vi "main_v1.vi"() -> ()   [LabVIEW 2020]
uses:
  <vilib>/Analysis/Matrix/Datatypes/RealMatrix.ctl
  C:/Program Files (x86)/National Instruments/LabVIEW 2020/examples/Instrument IO/Serial/support/Serial - Settings.ctl
  C:/Program Files (x86)/National Instruments/LabVIEW 2020/examples/Instrument IO/Serial/support/Serial - XON-XOFF Characters.ctl
  C:/Program Files (x86)/National Instruments/LabVIEW 2020/examples/Instrument IO/Serial/support/Serial - ASCII Characters.ctl
  <vilib>/Platform/TimedLoop/XDataNode/timing_clust.ctl
  <vilib>/Platform/TimedLoop/XDataNode/nitl_modes.ctl
  <vilib>/Platform/TimedLoop/XDataNode/wakeup.ctl
  <vilib>/Instr/_visa.llb/VISA Configure Serial Port (Instr).vi
  <vilib>/platform/TimedLoop/XDataNode/XDataNode.xnode
  <vilib>/Platform/TimedLoop/XDataNode/XDNodeRunTimeDep.lvlib
  <vilib>/Analysis/Matrix/NI_Matrix.lvlib
panel:
  out "Angle Plot":cluster{"Y":dbl[], "Y":dbl[]}[](graph)
  out "Z_GYRO":dbl(graph)
  out "Y_GYRO":dbl(graph)
  out "X_GYRO":dbl(graph)
  out "Z_ACC":dbl(graph)
  out "X_ACC":dbl(graph)
  out "Y_ACC":dbl(graph)
  out "Angular velocity after filtering":dbl
  out "pitch after filtering in degrees":dbl
  in  "Stop":bool
  in  "Read Count":u32=1000
  in  "?":bool
  in  "Termination Character":u8=10 format="%.0x"
  in  "End Write on Termination Character?":bool=TRUE
  in  "VISA resource name":refnum<visa-resource-name>="COM1"
  in  "XON/XOFF Characters":T1={"XON"=enum."DC1", "XOFF"=enum."DC3"}
  in  "Serial Settings":T3={"baud rate"=9600, "data bits"=8, "parity"=enum."None", "stop bits"=10, "flow control"=0} {"flow control" items=["None"=0, "XON/XOFF"=1, "RTS/CTS"=2, "DTR/DSR"=4]; "stop bits" items=["1.0"=10, "1.5"=15, "2.0"=20]; "data bits" min=5 max=8 step=1; "baud rate" items=["75"=75, "110"=110, "134"=134, "150"=150, "300"=300, "600"=600, "1200"=1200, "1800"=1800, "2400"=2400, "4800"=4800, "7200"=7200, "9600"=9600, "14400"=14400, "19200"=19200, "28800"=28800, "38400"=38400, "56000"=56000, "57600"=57600, "115200"=115200, "128000"=128000, "230400"=230400]}
  in  "End Read on Termination Character?":bool=TRUE
  out "Steady State Kalman Predictor Gain matrix":T4=[[-7.62521027355318e-05, 0.01032332398776421], [0.031126923690244213, -7.313941036650737e-06]]
  out "H Matrix":T4=[[0.0, 1.0], [1.0, 0.0]]
  out "G Matrix":T4=[[0.0001, -5e-09], [0.0, 0.0001]]
  out "F  Matrix":T4=[[1.0, -0.0001], [0.0, 1.0]]
  out "Q'=GQG' (Q scalar =1)":T4=[[1.0000000025e-08, -5e-13], [-5e-13, 1e-08]]
  out "State Predicted Estimate X^(k+1/k)":dbl[](array[numeric])=[-1.7557452195435928, 0.08364774980311916]
  out "Angular Velocity for Pitch":dbl(graph)
  out "Pitch Angle in degrees":dbl(graph)
  in  "Kalman Filter -> SWITCH OFF":bool=TRUE
  out "Raw X Gyro Velocity":dbl=-1.8293611669128778
  out "Raw accelerometer angle in degrees":dbl=-1.8293611669128778
  in  "X degrees  offset trim angle":dbl=-2.4999999999999982 min=-20.0 max=20.0 step=0.1
  in  "X offset trim gyro velocity":i16=60
  in  "Y offset trim gyro velocity":i16=-244
  out "Z_Acc":dbl=22.0 format="%.2f"
  out "Y_Acc":dbl=22.0 format="%.2f"
  out "X_Acc":dbl=22.0 format="%.2f"
  out "Z_Gyro_Rate":dbl=22.0 format="%.2f"
  out "X_Gyro_rate":dbl=22.0 format="%.2f"
  out "Y_Gyro_Rate":dbl=22.0 format="%.2f"
  # "Steady State Kalman Filter"
  # "-Prakhar Goel"
  # "Kalman Matrices"
  # "Serial Settings"
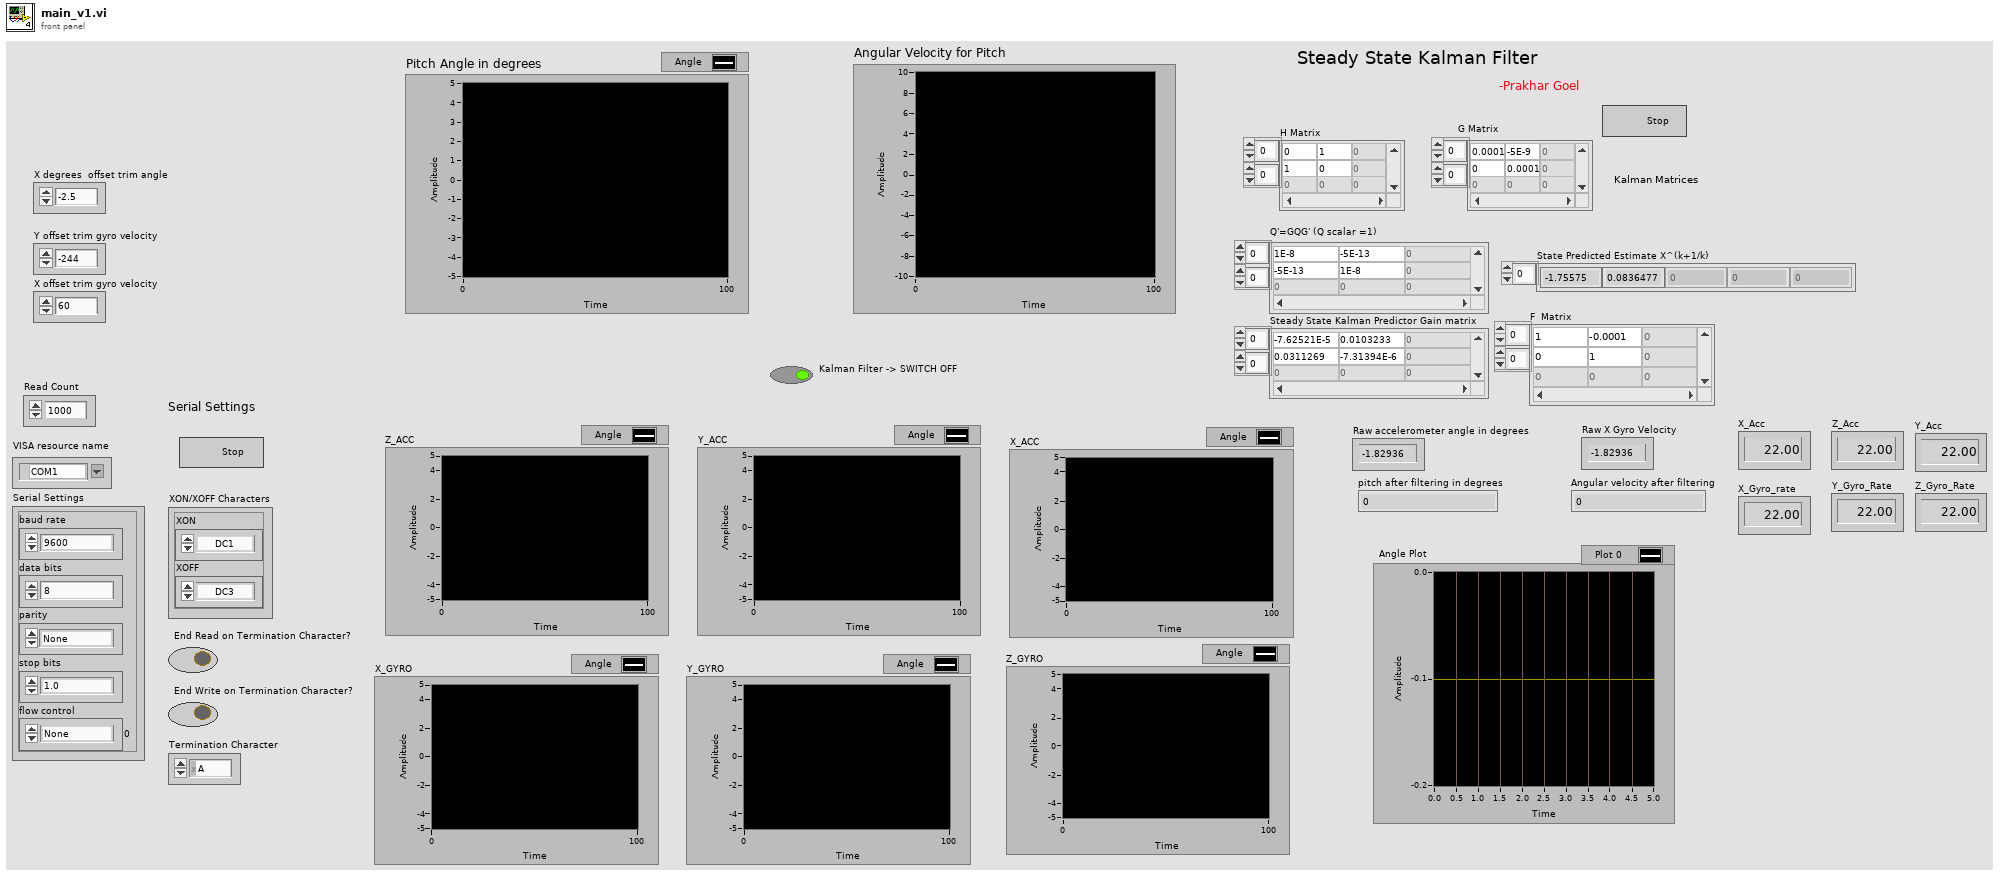
[diagram p1: front panel]
types:
  T1 = typedef "Serial - XON-XOFF Characters.ctl" = cluster{"XON":T2, "XOFF":T2}
  T2 = typedef "Serial - ASCII Characters.ctl" = enum16{"NUL", "SOH", "STX", "ETX", "EOT", "ENQ", "ACK", "BEL", "BS", "HT", "LF", "VT", "FF", "CR", "SO", "SI", "DLE", "DC1", "DC2", "DC3", "DC4", "NAK", "SYN", "ETB", "CAN", "EM", "SUB", "ESC", "FS", "GS", "RS", "US", "SP", "!", "\"", "#", "$", "%", "&", "'", "(", ")", "*", "+", ",", "- (-)", ".", "/", "0", "1", "2", "3", "4", "5", "6", "7", "8", "9", ":", ";", "<", "=", ">", "?", "@", "A", "B", "C", "D", "E", "F", "G", "H", "I", "J", "K", "L", "M", "N", "O", "P", "Q", "R", "S", "T", "U", "V", "W", "X", "Y", "Z", "[", "\\", "]", "^", "_", "`", "a", "b", "c", "d", "e", "f", "g", "h", "i", "j", "k", "l", "m", "n", "o", "p", "q", "r", "s", "t", "u", "v", "w", "x", "y", "z", "{", "|", "}", "~"}
  T3 = typedef "Serial - Settings.ctl" = cluster{"baud rate":u32, "data bits":u16, "parity":enum16{"None", "Odd", "Even", "Mark", "Space"}, "stop bits":u16, "flow control":u16}
  T4 = typedef "NI_Matrix.lvlib/RealMatrix.ctl" = dbl[][]
  T5 = typedef "XDNodeRunTimeDep.lvlib/timing_clust.ctl" = cluster{"Expected End [f-1]":u64, "Actual End [f-1]":u64, "Finished Late? [f-1]":bool, "Expected End [i-1]":u64, "Actual End [i-1]":u64, "Finished Late? [i-1]":bool, "Expected Start [i]":u64, "Actual Start [i]":u64, "Expected Start [f]":u64, "Actual Start [f]":u64, "Source Name":string, "Structure Name":string, "Period":i64, "Deadline":i64, "Offset":i64, "Start":i64, "Priority":i32, "Timeout":i32, "Mode":T6, "Wakeup Reason":T7, "Error":errorcluster, "Source Type":string, "Secondary Source Type":string, "Global End Time":u64, "Global Start Time":u64, "Frame Duration":u64, "Iteration Duration":u64, "Assigned CPU":i32, "I/O Scan Engine Mode":u32}
  T6 = typedef "XDNodeRunTimeDep.lvlib/nitl_modes.ctl" = enum32{"No Change", "Process missed periods, maintain original phase", "Discard missed periods, maintain original phase", "Process missed periods, ignore original phase", "Discard missed periods, ignore original phase"}
  T7 = typedef "XDNodeRunTimeDep.lvlib/wakeup.ctl" = enum32{"Normal", "Aborted", "Asynchronous wakeup", "Timing source error", "Timed loop error", "Timeout"}
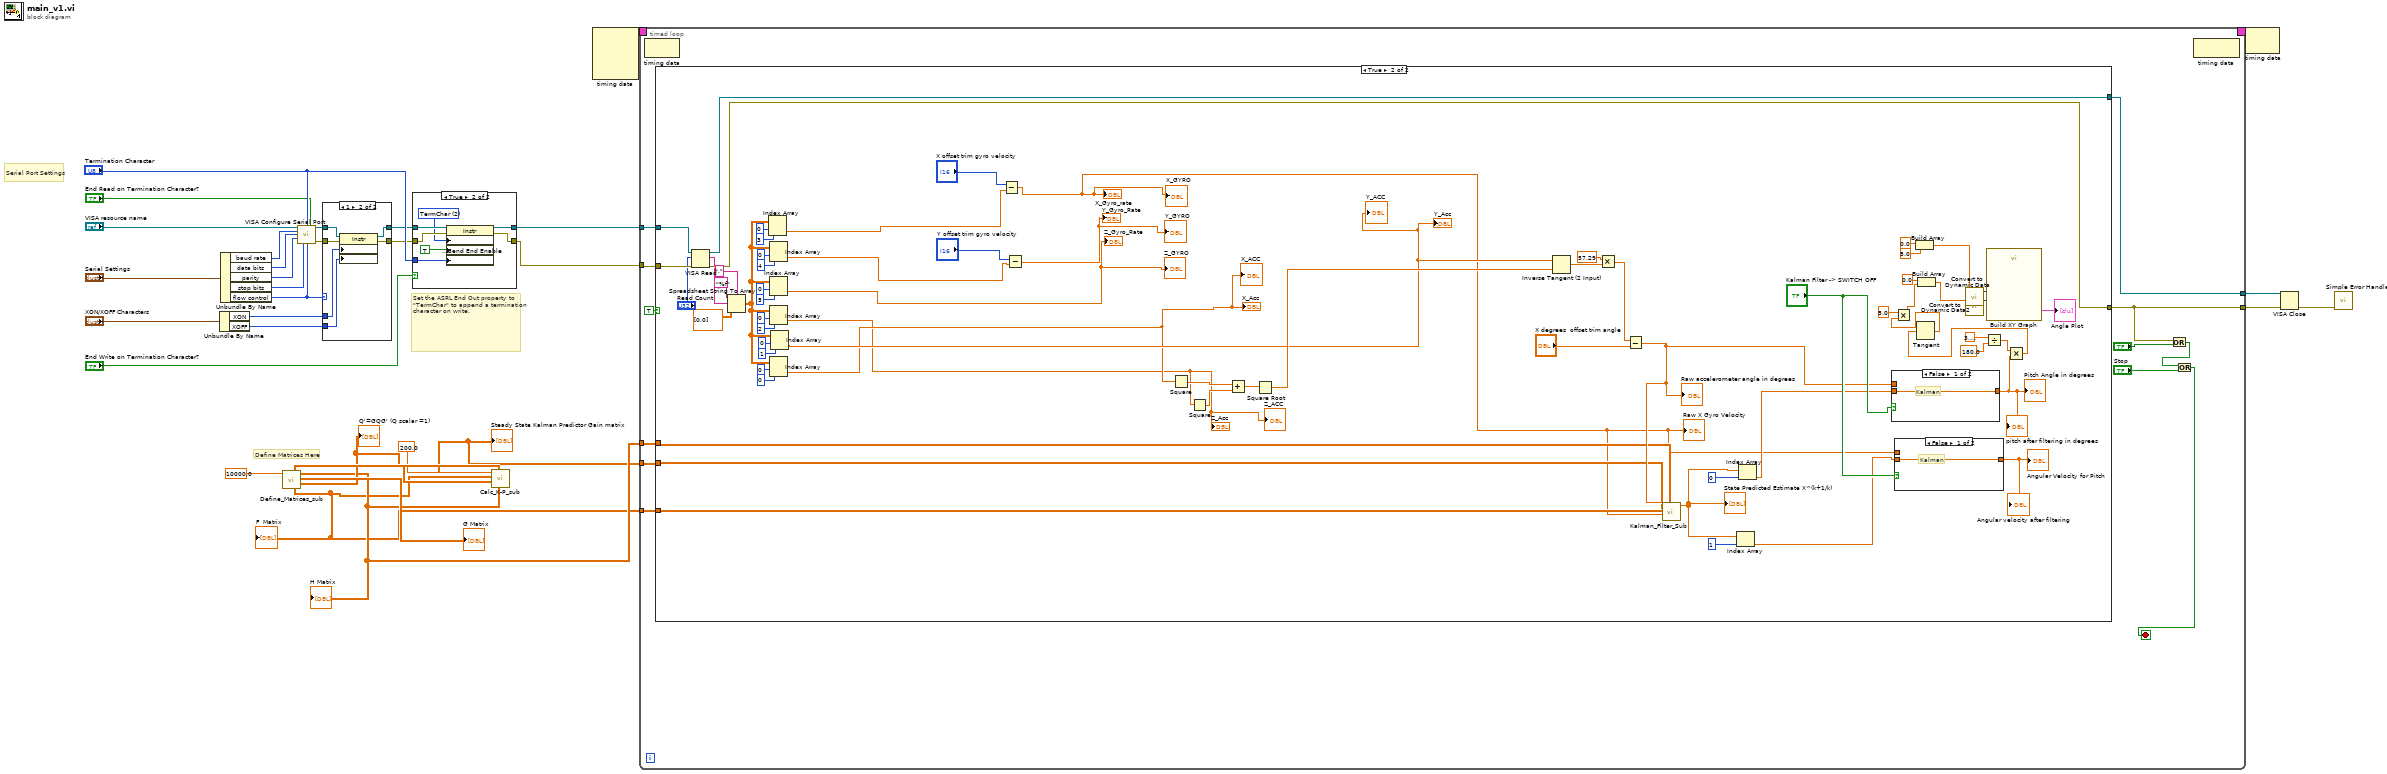
[diagram p0: block diagram]
diagram:
  # "Serial Port Settings"
  # "Set the ASRL End Out property to \"TermChar\" to append a termination character on write."
  # "Define Matrices Here"
  n1 = Unbundle By Name("XON/XOFF Characters") -> ("XON"=w17:T2, "XOFF"=w18:T2)
  n2 = Unbundle By Name("Serial Settings") -> ("baud rate"=w13:u32, "data bits"=w12:u16, "parity"=w11:enum16{"None", "Odd", "Even", "Mark", "Space"}, "stop bits"=w10:u16, "flow control"=w16:u16)
  n3 = call "Define_Matrices_sub.vi"("Sampling Freqauency (Hz)"=10000.0) -> ("Q = GQG'"=w26:T4, "G Matrix"=→"G Matrix":T4, "H Matrix"=w25:T4, "F  Matrix"=w24:T4, "R Matrix"=w28:T4)  [unwired: 6 in]
  "Q'=GQG' (Q scalar =1)" <- w26
  "F  Matrix" <- w24
  "H Matrix" <- w25
  n4 = call-poly "VISA Configure Serial Port"("VISA resource name"="VISA resource name", "termination char\n(0xA = '\\n' = LF)"="Termination Character", "Enable Termination\nChar (T)"="End Read on Termination Character?", "baud rate (9600)"=w13, "data bits (8)"=w12, "parity (0:none)"=w11, "stop bits (10: 1 bit)"=w10, "flow control (0:none)"=w16) -> ("VISA resource name out"=w9:refnum<visa-resource-name>, "error out"=w8:errorcluster)  [unwired: 2 in, 4 out]
  n5 = case shown="1" w16 {
    tunnel: [w33 w40] -> w19
    tunnel: [w34 w39] -> w20
    tunnel: w8 -> [w33 w38]
    tunnel: w9 -> [w34 w37]
    tunnel: w17 -> [_ w36]
    tunnel: w18 -> [_ w35]
    frame Default {
    }
    frame 1 {
      n6 = property class="Instr"(reference=w37, error in=w38, "Serial Settings:Flow Control XON Character"=w36, "Serial Settings:Flow Control XOFF Character"=w35) -> (reference out=w39:refnum<visa-resource-name>, error out=w40:errorcluster)
    }
  }
  n7 = case shown="True" "End Write on Termination Character?" {
    tunnel: w20 -> [w41 w49]
    tunnel: w19 -> [w42 w48]
    tunnel: [w41 w47] -> w4
    tunnel: [w42 w46] -> w5
    tunnel: "Termination Character" -> [_ w44]
    frame False {
    }
    frame True {
      w45 = u16 2 items=["None", "LastBit", "TermChar", "Break"] ("Serial Settings:Serial End Mode for Writes")
      n8 = property class="Instr"(reference=w49, error in=w48, "Serial Settings:End Mode for Writes"=w45, "Message Based Settings:Send End Enable"=TRUE, "Message Based Settings:Termination Character"=w44) -> (reference out=w47:refnum<visa-resource-name>, error out=w46:errorcluster)
    }
  }
  n9 = call "Calc_K-P_sub.vi"("H Matrix"=w25, "R Matrix"=w28, "Q'=GQG' (Q scalar =1)"=w26, "F  Matrix"=w24, "Number of iterations"=200.0 ("Sampling Freqauency (Hz)")) -> ("Steady State Kalman Predictor Gain matrixx"=w23:T4)  [unwired: 4 in, 2 out]
  "Steady State Kalman Predictor Gain matrix" <- w23
  n10 = node-c288() -> (w32:T5)  [unwired: 4 in]
  n11 = timed-loop {
    timing: w32 -> [_]
    timing-out: [_] -> w31
    tunnel: w25 -> [w61]
    tunnel: w24 -> [w60]
    tunnel: w23 -> [w59]
    tunnel: w5 -> [w58]
    tunnel: w4 -> [w57]
    tunnel: [w56] -> w3
    tunnel: [w54] -> w2
    stop <- w50 stop-if-true
    n12 = node-c288() -> ()  [unwired: 1 in, 1 out]
    n13 = case shown="True" TRUE {
      tunnel: w61 -> [_ w112]
      tunnel: w60 -> [_ w111]
      tunnel: w59 -> [_ w110]
      tunnel: w58 -> [w62 w109]
      tunnel: w57 -> [w63 w108]
      tunnel: [w63 w107] -> w56
      tunnel: [w62 w106] -> w54
      frame False {
      }
      frame True {
        n14 = VISA Read(VISA resource name=w108, byte count="Read Count", error in (no error)=w109) -> (VISA resource name out=w107:refnum<visa-resource-name>, read buffer=w104:string, error out=w106:errorcluster)  [unwired: 1 out]
        n15 = Spreadsheet String To Array(delimiter (Tab)=",", format string="%f", spreadsheet string=w104, array type (2D Dbl)=dbl[][] [[0.0]]) -> (array=w103:dbl[][])
        n16 = Index Array(array=w103, index (row)=0, index (col)=3 ("disabled index (col)")) -> (element=w87:dbl)
        n17 = Index Array(array=w103, index (row)=0, index (col)=5 ("disabled index (col)")) -> (element=→"Z_Gyro_Rate" →"Z_GYRO":dbl)
        n18 = Index Array(array=w103, index (row)=0, index (col)=4 ("disabled index (col)")) -> (element=w86:dbl)
        n19 = Index Array(array=w103, index (row)=0, index (col)=2 ("disabled index (col)")) -> (element=w83:dbl)
        "Z_Acc" <- w83
        "Z_ACC" <- w83
        n20 = Index Array(array=w103, index (row)=0, index (col)=0 ("disabled index (col)")) -> (element=w84:dbl)
        "X_Acc" <- w84
        "X_ACC" <- w84
        n21 = Index Array(array=w103, index (row)=0, index (col)=1 ("disabled index (col)")) -> (element=w85:dbl)
        "Y_Acc" <- w85
        "Y_ACC" <- w85
        n22 = Subtract(x="X offset trim gyro velocity", y=w87) -> (x-y=w82:dbl)
        "X_Gyro_rate" <- w82
        "Raw X Gyro Velocity" <- w82
        "X_GYRO" <- w82
        n23 = Subtract(x="Y offset trim gyro velocity", y=w86) -> (x-y=→"Y_Gyro_Rate" →"Y_GYRO":dbl)
        n24 = Square(x=w84) -> (x^2=w123:dbl)
        n25 = Square(x=w83) -> (x^2=w122:dbl)
        n26 = Add(x=w123, y=w122) -> (x+y=w124:dbl)
        n27 = Square Root(x=w124) -> (sqrt(x)=w121:dbl)
        n28 = Inverse Tangent (2 Input)(1:w121, 2:w85) -> (0:w125:dbl)
        n29 = Multiply(x=57.29, y=w125) -> (x*y=w128:dbl)
        n30 = Subtract(x=w128, y="X degrees  offset trim angle") -> (x-y=w113:dbl)
        "Raw accelerometer angle in degrees" <- w113
        n31 = call "Kalman_Filter_Sub.vi"("F  Matrix"=w111, "H Matrix"=w112, "Gyro"=w82, "Steady State Kalman Predictor Gain matrix"=w110, "accelerometer angle"=w113) -> ("State Predicted Estimate X^(k+1/k)"=w114:dbl[])  [unwired: 6 in]
        "State Predicted Estimate X^(k+1/k)" <- w114
        n32 = Index Array(array=w114, index=1) -> (element=w115:dbl)
        n33 = Index Array(array=w114, index=0) -> (element=w116:dbl)
        n34 = case shown="False" "Kalman Filter -> SWITCH OFF" {
          tunnel: w113 -> [_ w134]
          tunnel: [w133 w134] -> w68
          tunnel: w116 -> [w133 _]
          frame False {
            # "Kalman"
          }
          frame True {
            # "Accelerometer\nangle on its own"
          }
        }
        "Pitch Angle in degrees" <- w68
        "pitch after filtering in degrees" <- w68
        n35 = case shown="False" "Kalman Filter -> SWITCH OFF" {
          tunnel: w82 -> [_ w132]
          tunnel: [w131 w132] -> w119
          tunnel: w115 -> [w131 _]
          frame False {
            # "Kalman"
          }
          frame True {
            # "Accelerometer\nangle on its own"
          }
        }
        "Angular Velocity for Pitch" <- w119
        "Angular velocity after filtering" <- w119
        n36 = Build Array(0.0 ("element"), 5.0 ("element")) -> (w76:dbl[])
        n37 = call "Convert to Dynamic Data"("Array"=w76) -> ("Dynamic Data Type"=w75:dynamicdata)  [unwired: 3 in]
        n38 = Divide(x=3.141592653589793, y=180.0) -> (x/y=w69:dbl)
        n39 = Multiply(x=w69, y=w68) -> (x*y=w67:dbl)
        n40 = Tangent(1:w67) -> (0:w66:dbl)
        n41 = Multiply(x=5.0, y=w66) -> (x*y=w64:dbl)
        n42 = Build Array(0.0 ("element"), w64) -> (w73:dbl[])
        n43 = call "Convert to Dynamic Data2"("Array"=w73) -> ("Dynamic Data Type"=w72:dynamicdata)  [unwired: 3 in]
        n44 = call "Build XY Graph"("Y Input"=w72, "X Input"=w75) -> ("XY Graph"=→"Angle Plot":cluster{"X":dbl[], "Y":dbl[]}[])  [unwired: 8 in, 1 out]
      }
    }
    n45 = Or(x=w54, y="?") -> (x .or. y?=w52:bool)
    n46 = Or(x=w52, y="Stop") -> (x .or. y?=w50:bool)
    n47 = node-c288() -> ()  [unwired: 1 in, 1 out]
  }
  n48 = node-c288(w31) -> ()  [unwired: 1 out]
  n49 = VISA Close(VISA resource name=w3, error in (no error)=w2) -> (error out=w1:errorcluster)
  n50 = call <vilib>:"Simple Error Handler.vi"("error in (no error)"=w1) -> ()  [unwired: 4 in, 5 out]
